vi "SV verifier.vi"(8 "error in (no error)":errorcluster, 11 "SV name in":string) -> (0 "error out":errorcluster, 3 "Refnum out":refnum<k21>)   [LabVIEW 2020, in "TALOS.lvlib" / "Father of all uServices.lvlib" / "Father of all uServices.lvclass"]
uses:
  Father of all uServices.lvclass
  Classes/Circus Shared Variables/Circus Shared Variables.lvclass/Circus Shared Variables.ctl
  Ancestor/Ancestor/Ancestor.lvclass/Ancestor.ctl
  Support VIs/Substitute Error.vi
  Support VIs/Generate Error.vi
  FGV/Error Memory/Get Error Description.vi
  Support VIs/Get PC name.vi
  Ancestor/Ancestor/Read ID.vi
  Support VIs/Get Class Name.vi
  <vilib>/Utility/error.llb/Clear Errors.vi
  FGV/Error Memory/Error Memory Core.vi
  <vilib>/AdvancedString/Delimited String to 1D String Array.vi
  Support VIs/Circus Root Path.vi
  FGV/Error Memory/Error Crt Lvl checker.vi
  FGV/Error Memory/Error Memory Core.vi/40c8088d-b597-4017-91af-faa98e00292e.vi
  FGV/Error Memory/Error Memory Core.vi/d4a3ab98-063c-4e44-b43d-fbdcfe6c2be2.vi
  Support VIs/Global Memory.vi
  <vilib>/Utility/LVClass/Get LV Class Name.vi
  Support VIs/Is in Packed Library.vi
  Support VIs/TALOS Root path.vi
  Support VIs/Read CSV worksheet.vi
  Support VIs/Global Constants.vi
  <vilib>/Utility/error.llb/General Error Handler.vi
  Support VIs/Error Log.vi
  Ancestor/Ancestor/Ancestor.lvclass
  <vilib>/Comparison/Equal/Equal Functor/Equal Functor.lvclass
  Father of all uServices.lvclass/Father of all uServices.ctl
  Classes/Circus Shared Variables/Circus Shared Variables.lvclass
  TALOS.lvlib
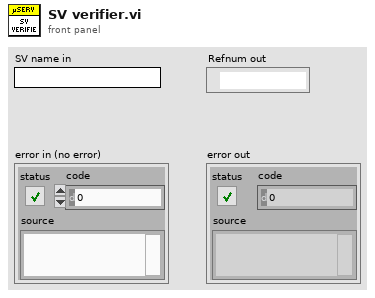
[diagram p1: front panel]
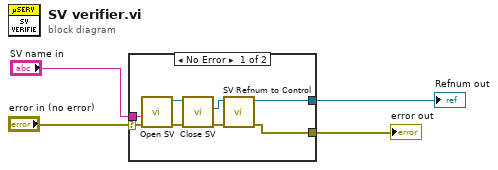
[diagram p0: block diagram]
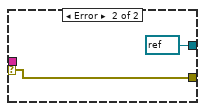
[diagram p2: hidden frame]
diagram:
  n1 = case shown="No Error" "error in (no error)" {
    selector: "error in (no error)" -> [w6 w13]
    tunnel: [w12 w13] -> w4
    tunnel: [w11 refnum<k21> refnum ("Shared Variable Control Out")] -> w3
    tunnel: "SV name in" -> [w7 _]
    frame No Error {
      n2 = call "Open SV.vi"("error in (no error)"=w6, "SV Name"=w7) -> ("error out"=w5:errorcluster, "AEgIS Shared Variables out"=w8:refnum<class "Circus Shared Variables.lvclass">)  [unwired: 8 in]
      n3 = call "Close SV.vi"("error in (no error)"=w5, "AEgIS Shared Variables in"=w8) -> ("error out"=w9:errorcluster, "SV"=w10:refnum<k21>)  [unwired: 7 in, 1 out]
      n4 = call "SV Refnum to Control.vi"("error in (no error)"=w9, "shared variable refnum in"=w10) -> ("error out"=w12:errorcluster, "Shared Variable Control Out"=w11:refnum<k21>)  [unwired: 8 in]
    }
    frame Error {
    }
  }
  "error out" <- w4
  "Refnum out" <- w3
